vi "Configure UART.vi"(8 "error in (no error)":errorcluster, 9 "UART configuration":T1 {"flow control" items=["none", "rts", "cts", "rts/cts"]; "stop bits" items=["1", "1.5", "2"]; "parity" items=["none", "even", "odd"]}, 10 "hardware interface index":u16, 11 "PLBB in":refnum<class "PL BlackBox Modbus Client.lvclass">) -> (0 "error out":errorcluster, 3 "PLBB out":refnum<class "PL BlackBox Modbus Client.lvclass">)   [LabVIEW 2015, in "PL BlackBox Modbus Client.lvclass"]
doc: "Configures the UART."
uses:
  PL BlackBox Modbus Client.lvclass
  <vilib>/plasmapper/PL Modbus Client/PL Modbus Client.lvclass
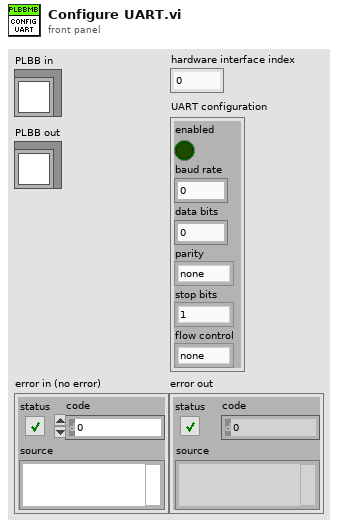
[diagram p1: front panel]
types:
  T1 = cluster{"enabled":bool, "baud rate":u32, "data bits":u16, "parity":u16, "stop bits":u16, "flow control":u16}
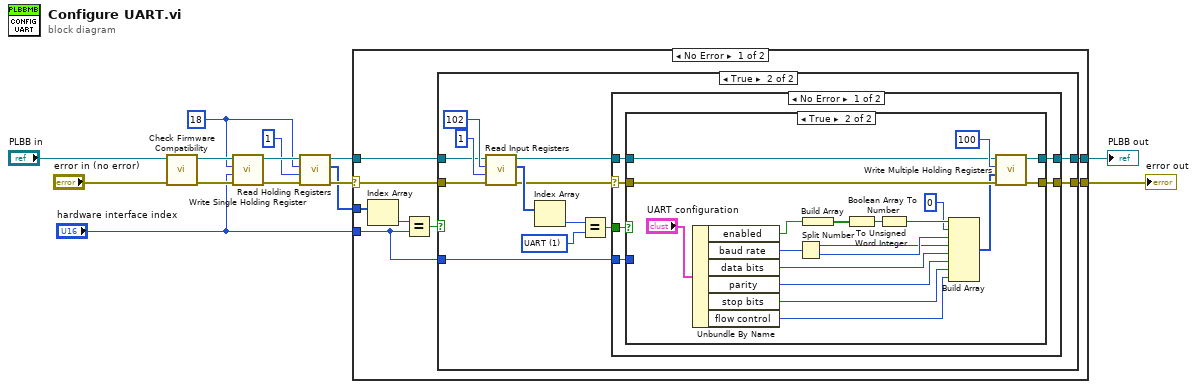
[diagram p0: block diagram]
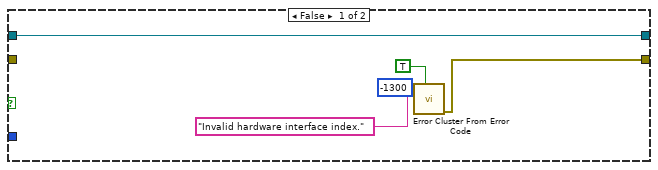
[diagram p2: hidden frame]
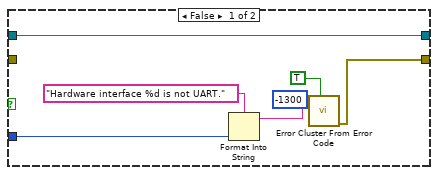
[diagram p3: hidden frame]
diagram:
  w6 = u16 18 ("address")
  n1 = call-dynamic "Check Firmware Compatibility.vi"("error in (no error)"="error in (no error)", "PLBB in"="PLBB in") -> ("error out"=w9:errorcluster, "PLBB out"=w10:refnum<class "PL BlackBox Modbus Client.lvclass">)  [unwired: 8 in]
  n2 = call <vilib>:"Write Single Holding Register.vi"("error in (no error)"=w9, "value"="hardware interface index", "address"=w6, "MODBUS in"=w10) -> ("error out"=w5:errorcluster, "MODBUS out"=w8:refnum<class "PL BlackBox Modbus Client.lvclass">)  [unwired: 6 in]
  n3 = call <vilib>:"Read Holding Registers.vi"("error in (no error)"=w5, "number of holding registers"=u16 1 ("address"), "address"=w6, "MODBUS in"=w8) -> ("error out"=w4:errorcluster, "values"=w2:u16[], "MODBUS out"=w3:refnum<class "PL BlackBox Modbus Client.lvclass">)  [unwired: 5 in]
  n4 = case shown="No Error" w4 {
    selector: w4 -> [w16 w75]
    tunnel: [w22 w75] -> w14
    tunnel: [w21 w76] -> w13
    tunnel: w3 -> [w17 w76]
    tunnel: w2 -> [w20 _]
    tunnel: "hardware interface index" -> [w15 _]
    frame No Error {
      n5 = Index Array(array=w20) -> (element=w19:u16)  [unwired: 1 in]
      n6 = Equal?(x=w19, y=w15) -> (x = y?=w18:bool)
      n7 = case shown="True" w18 {
        tunnel: [w23 w29] -> w22
        tunnel: [w27 w30] -> w21
        tunnel: w17 -> [w27 w38]
        tunnel: w16 -> [_ w37]
        tunnel: w15 -> [_ w28]
        frame False {
          n8 = call <vilib>:"Error Cluster From Error Code.vi"("show call chain? (False)"=TRUE, "error message (\"\")"="Invalid hardware interface index." ("error message (\"\")"), "error code (0)"=-1300) -> ("error out"=w23:errorcluster)  [unwired: 6 in]
        }
        frame True {
          w34 = u16 1 items=["Unknown", "UART", "Network interface", "Ethernet", "Wi-Fi"] ("type")
          n9 = call <vilib>:"Read Input Registers.vi"("error in (no error)"=w37, "number of input registers"=u16 1 ("address"), "address"=u16 102, "MODBUS in"=w38) -> ("error out"=w32:errorcluster, "values"=w36:u16[], "MODBUS out"=w31:refnum<class "PL BlackBox Modbus Client.lvclass">)  [unwired: 5 in]
          n10 = Index Array(array=w36) -> (element=w35:u16)  [unwired: 1 in]
          n11 = Equal?(x=w35, y=w34) -> (x = y?=w33:bool)
          n12 = case shown="No Error" w32 {
            selector: w32 -> [w44 w73]
            tunnel: w33 -> [w46 _]
            tunnel: [w41 w74] -> w30
            tunnel: w31 -> [w45 w74]
            tunnel: [w42 w73] -> w29
            tunnel: w28 -> [w43 _]
            frame No Error {
              n13 = case shown="True" w46 {
                tunnel: w45 -> [w47 w68]
                tunnel: w44 -> [_ w67]
                tunnel: w43 -> [w50 _]
                tunnel: [w48 w71] -> w42
                tunnel: [w47 w72] -> w41
                frame False {
                  n14 = Format Into String(format string="Hardware interface %d is not UART." ("error message (\"\")"), w50) -> (resulting string=w49:string)  [unwired: 2 in, 1 out]
                  n15 = call <vilib>:"Error Cluster From Error Code.vi"("show call chain? (False)"=TRUE, "error message (\"\")"=w49, "error code (0)"=-1300) -> ("error out"=w48:errorcluster)  [unwired: 6 in]
                }
                frame True {
                  n16 = Unbundle By Name("UART configuration") -> ("enabled"=w63:bool, "baud rate"=w66:u32, "data bits"=w59:u16, "parity"=w58:u16, "stop bits"=w57:u16, "flow control"=w56:u16)
                  n17 = Split Number(x=w66) -> (hi(x)=w60:u16, lo(x)=w61:u16)
                  n18 = Build Array(w63) -> (w64:bool[])
                  n19 = Boolean Array To Number(Boolean array=w64) -> (number=w65:u32)
                  n20 = To Unsigned Word Integer(number=w65) -> (unsigned 16bit integer=w62:u16)
                  n21 = Build Array(w62, u16 0 ("element"), w61, w60, w59, w58, w57, w56) -> (w55:u16[])
                  n22 = call <vilib>:"Write Multiple Holding Registers.vi"("error in (no error)"=w67, "values"=w55, "address"=u16 100, "MODBUS in"=w68) -> ("error out"=w71:errorcluster, "MODBUS out"=w72:refnum<class "PL BlackBox Modbus Client.lvclass">)  [unwired: 6 in]
                }
              }
            }
            frame Error {
            }
          }
        }
      }
    }
    frame Error {
    }
  }
  "error out" <- w14
  "PLBB out" <- w13
